vi "motor CNTR & CNFG.vi"(0 "FPGA VI Reference":refnum<k20>, 1 "speed duty cycle":dbl, 3 "Motor Brake":bool, 4 "Motor select":T2, 5 "Error In":errorcluster, 7 "Motor period":i64, 8 "Function":T1, 9 "Motor.enable_divider":bool, 11 "Motor.divider":fxp<+,4,4>) -> (14 "FPGA VI Reference Out":refnum<k20>, 17 "Frequence":dbl, 19 "error out":errorcluster)   [LabVIEW 2019, in "Motor single.lvclass"]
uses:
  Motor single.lvclass
  motor enum(FPGA).ctl
  motor control & config.ctl
  <vilib>/Utility/error.llb/Error Cluster From Error Code.vi
  <vilib>/rvi/errors/niLvFpgaAdjustHostInterfaceError.vi
  <vilib>/rvi/interface/nirviReadWriteControl/nirviReadWriteControl.xnode
  NiFpgaLv.dll
  <vilib>/rvi/interface/Simulation/niFpgaSimulationCallBeginRW.vi
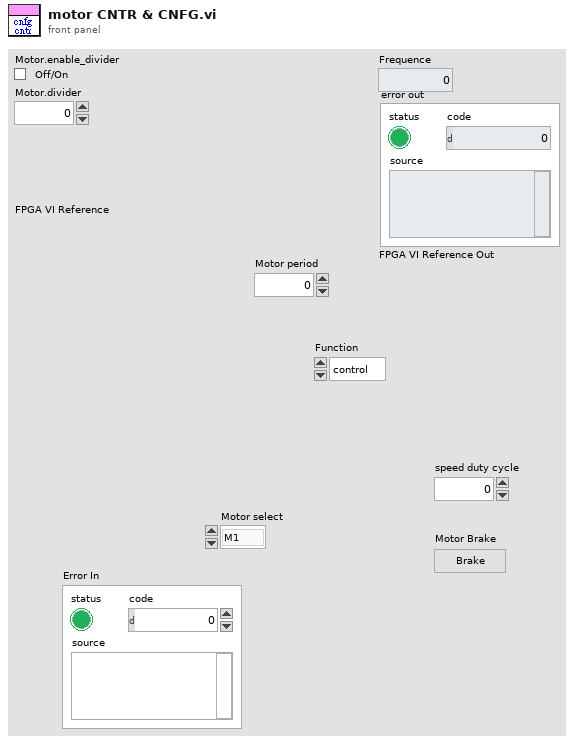
[diagram p1: front panel]
types:
  T1 = typedef "Motor single.lvclass/motor control & config.ctl" = enum16{"control", "config"}
  T2 = typedef "Motor single.lvclass/motor enum(FPGA).ctl" = enum16{"M1", "M2", "M3", "M4"}
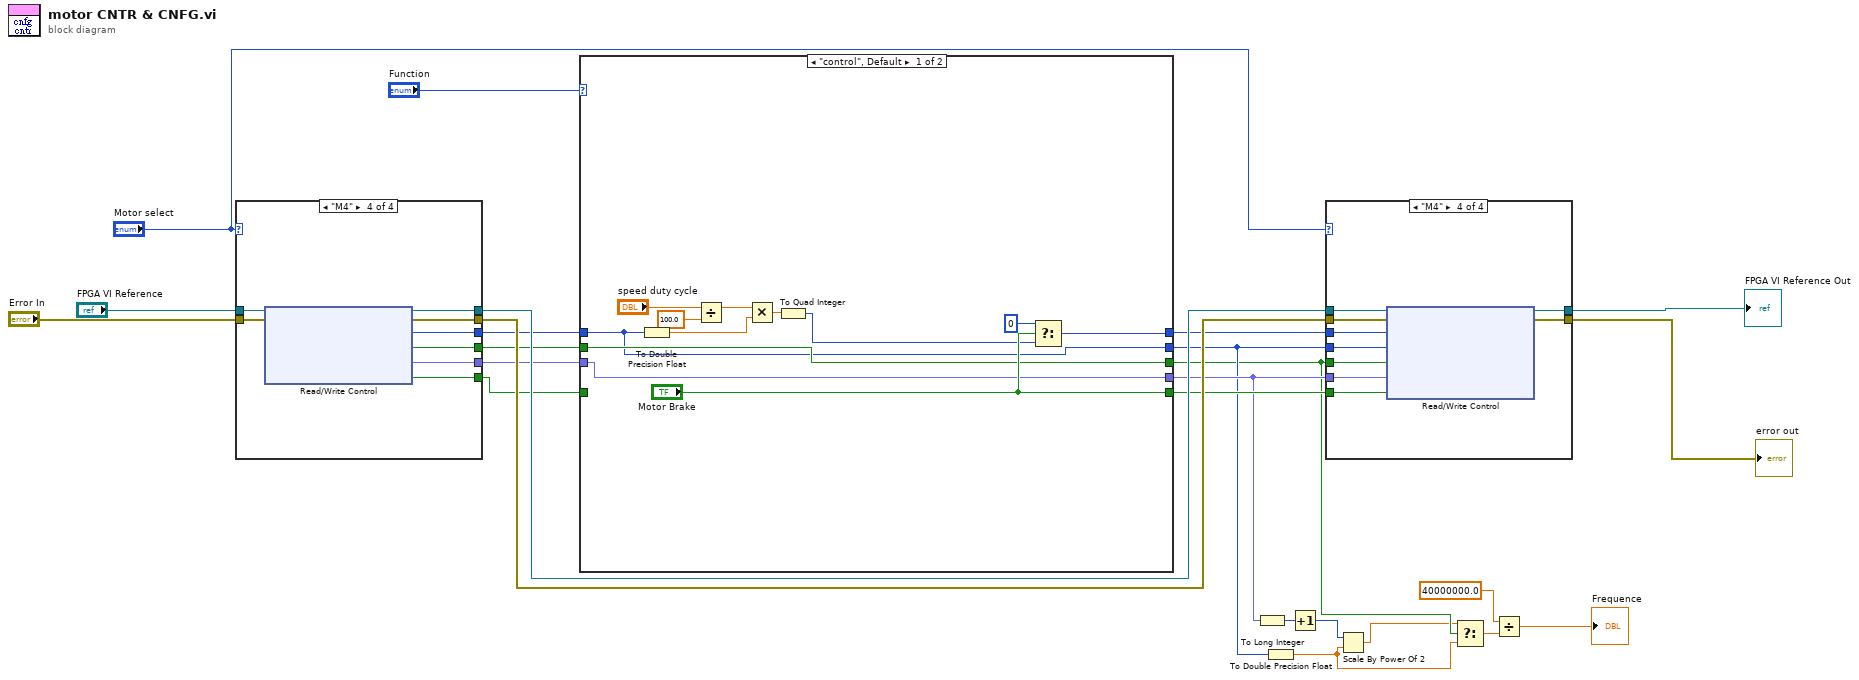
[diagram p0: block diagram]
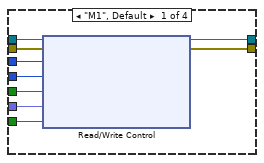
[diagram p2: hidden frame]
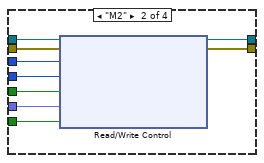
[diagram p3: hidden frame]
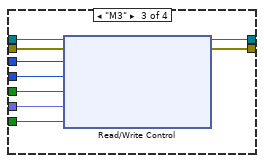
[diagram p4: hidden frame]
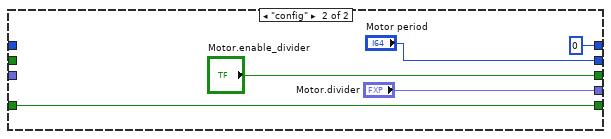
[diagram p5: hidden frame]
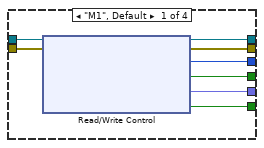
[diagram p6: hidden frame]
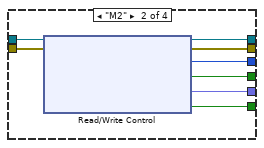
[diagram p7: hidden frame]
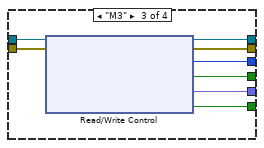
[diagram p8: hidden frame]
diagram:
  n1 = case shown="\"M4\"" "Motor select" {
    tunnel: "FPGA VI Reference" -> [w32 w35 w48 w56]
    tunnel: "Error In" -> [w31 w34 w47 w55]
    tunnel: [w30 w36 w46 w54] -> w19
    tunnel: [w29 w37 w45 w53] -> w20
    tunnel: [w28 w40 w44 w50] -> w18
    tunnel: [w27 w39 w43 w51] -> w14
    tunnel: [w26 w38 w42 w52] -> w15
    tunnel: [w25 w33 w41 w49] -> w13
    frame "M1", Default {
      n2 = xnode "Read/Write Control"("FPGA VI Reference In"=w32, "error in"=w31) -> ("FPGA VI Reference Out"=w29:refnum<k20>, "error out"=w30:errorcluster, "Motor1.periode"=w28:i64, "Motor1.enable_divider"=w27:bool, "Motor1.divider"=w26:fxp<+,4,4>, "Motor1.brake"=w25:bool)
    }
    frame "M2" {
      n3 = xnode "Read/Write Control"("FPGA VI Reference In"=w35, "error in"=w34) -> ("FPGA VI Reference Out"=w37:refnum<k20>, "error out"=w36:errorcluster, "Motor2.periode"=w40:i64, "Motor2.enable_divider"=w39:bool, "Motor2.divider"=w38:fxp<+,4,4>, "Motor2.brake"=w33:bool)
    }
    frame "M3" {
      n4 = xnode "Read/Write Control"("FPGA VI Reference In"=w48, "error in"=w47) -> ("FPGA VI Reference Out"=w45:refnum<k20>, "error out"=w46:errorcluster, "Motor3.periode"=w44:i64, "Motor3.enable_divider"=w43:bool, "Motor3.divider"=w42:fxp<+,4,4>, "Motor3.brake"=w41:bool)
    }
    frame "M4" {
      n5 = xnode "Read/Write Control"("FPGA VI Reference In"=w56, "error in"=w55) -> ("FPGA VI Reference Out"=w53:refnum<k20>, "error out"=w54:errorcluster, "Motor4.periode"=w50:i64, "Motor4.enable_divider"=w51:bool, "Motor4.divider"=w52:fxp<+,4,4>, "Motor4.brake"=w49:bool)
    }
  }
  n6 = case shown="\"control\", Default" "Function" {
    tunnel: w18 -> [w59 _]
    tunnel: ["Motor Brake" w73] -> w17
    tunnel: [w62 i64 0 ("t")] -> w16
    tunnel: w15 -> [w61 _]
    tunnel: [w61 "Motor.divider"] -> w12
    tunnel: w14 -> [w60 _]
    tunnel: [w60 "Motor.enable_divider"] -> w3
    tunnel: [w59 "Motor period"] -> w11
    tunnel: w13 -> [_ w73]
    frame "control", Default {
      n7 = To Double Precision Float(number=w59) -> (double precision float=w67:dbl)
      n8 = Divide(x="speed duty cycle", y=100.0) -> (x/y=w58:dbl)
      n9 = Multiply(x=w58, y=w67) -> (x*y=w66:dbl)
      n10 = To Quad Integer(1:w66) -> (0:w64:i64)
      n11 = Select(t=i64 0, s="Motor Brake", f=w64) -> (s? t:f=w62:i64)
    }
    frame "config" {
    }
  }
  n12 = To Long Integer(number=w12) -> (32bit integer=w10:i32)
  n13 = To Double Precision Float(number=w11) -> (double precision float=w1:dbl)
  n14 = Increment(x=w10) -> (x+1=w9:i32)
  n15 = case shown="\"M4\"" "Motor select" {
    tunnel: w20 -> [w82 w84 w98 w106]
    tunnel: w19 -> [w81 w85 w97 w107]
    tunnel: [w80 w83 w100 w109] -> w6
    tunnel: [w79 w91 w99 w108] -> w5
    tunnel: w17 -> [w78 w90 w92 w101]
    tunnel: w16 -> [w77 w86 w96 w105]
    tunnel: w12 -> [w76 w89 w93 w102]
    tunnel: w3 -> [w75 w88 w94 w103]
    tunnel: w11 -> [w74 w87 w95 w104]
    frame "M1", Default {
      n16 = xnode "Read/Write Control"("FPGA VI Reference In"=w82, "error in"=w81, "Motor1.speed"=w77, "Motor1.periode"=w74, "Motor1.enable_divider"=w75, "Motor1.divider"=w76, "Motor1.brake"=w78) -> ("FPGA VI Reference Out"=w79:refnum<k20>, "error out"=w80:errorcluster)
    }
    frame "M2" {
      n17 = xnode "Read/Write Control"("FPGA VI Reference In"=w84, "error in"=w85, "Motor2.speed"=w86, "Motor2.periode"=w87, "Motor2.enable_divider"=w88, "Motor2.divider"=w89, "Motor2.brake"=w90) -> ("FPGA VI Reference Out"=w91:refnum<k20>, "error out"=w83:errorcluster)
    }
    frame "M3" {
      n18 = xnode "Read/Write Control"("FPGA VI Reference In"=w98, "error in"=w97, "Motor3.speed"=w96, "Motor3.periode"=w95, "Motor3.enable_divider"=w94, "Motor3.divider"=w93, "Motor3.brake"=w92) -> ("FPGA VI Reference Out"=w99:refnum<k20>, "error out"=w100:errorcluster)
    }
    frame "M4" {
      n19 = xnode "Read/Write Control"("FPGA VI Reference In"=w106, "error in"=w107, "Motor4.speed"=w105, "Motor4.periode"=w104, "Motor4.enable_divider"=w103, "Motor4.divider"=w102, "Motor4.brake"=w101) -> ("FPGA VI Reference Out"=w108:refnum<k20>, "error out"=w109:errorcluster)
    }
  }
  "error out" <- w6
  "FPGA VI Reference Out" <- w5
  n20 = Scale By Power Of 2(n=w9, x=w1) -> (x*2^n=w2:dbl)
  n21 = Select(t=w2, s=w3, f=w1) -> (s? t:f=w4:dbl)
  n22 = Divide(x=40000000.0, y=w4) -> (x/y=→"Frequence":dbl)
